vi "lsl destroy continuous resolver.vi"(8 "error in (no error)":errorcluster, 11 "res":cluster{}) -> (0 "error out":errorcluster, 3 "res out":cluster{})   [LabVIEW 2016, in "Lab Streaming Layer.lvlib"]
doc: "extern LIBLSL_C_API void lsl_destroy_continuous_resolver(lsl_continuous_resolver res);"
uses:
  Lab Streaming Layer.lvlib
  liblsl-LabVIEW-master/liblsl-LabVIEW-master/lsl.dll
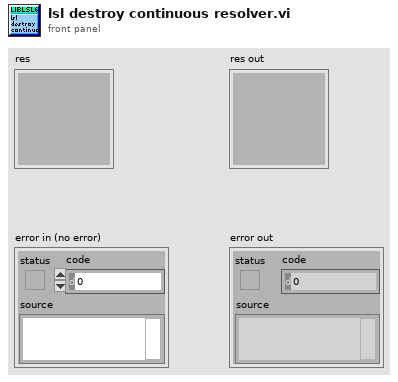
[diagram p1: front panel]
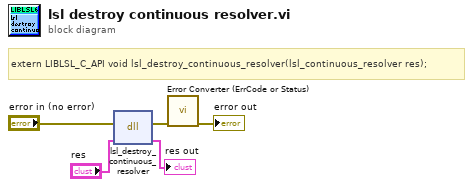
[diagram p0: block diagram]
diagram:
  # "extern LIBLSL_C_API void lsl_destroy_continuous_resolver(lsl_continuous_resolver res);"
  n1 = dll-call lib="E:/LabStreamingLayer/liblsl-LabVIEW-master/liblsl-LabVIEW-master/lsl.dll" fn="lsl_destroy_continuous_resolver"(error in="error in (no error)", "res"="res") -> (error out=w2:errorcluster, "res"=→"res out":cluster{})  [unwired: 3 in, 1 out]
  n2 = call "Error Converter (ErrCode or Status).vi"("error in (no error)"=w2) -> ("error out"=→"error out":errorcluster)  [unwired: 10 in]
